vi "Write LNA Status.vi"(10 "LNA Status":T1, 11 "Test LNA in":refnum<class "TestLNA.lvclass">) -> (3 "Test LNA out":refnum<class "TestLNA.lvclass">)   [LabVIEW 2016, in "TestLNA.lvlib" / "TestLNA.lvclass"]
uses:
  TestLNA.lvclass
  TestLNA.lvclass/TestLNA.ctl
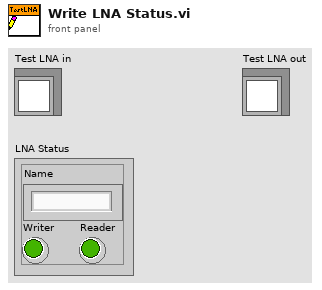
[diagram p1: front panel]
types:
  T1 = cluster{"Name":string, "Writer":bool, "Reader":bool}
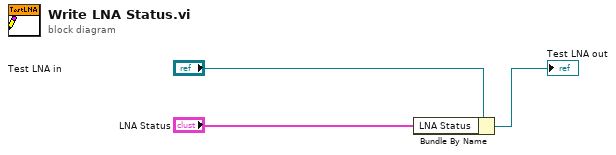
[diagram p0: block diagram]
diagram:
  n1 = Bundle By Name(cluster="Test LNA in", "LNA Status"="LNA Status") -> (→"Test LNA out":refnum<class "TestLNA.lvclass">)
